vi "Required Buffer Size.vi"(8 "error in (no error)":errorcluster, 11 "Transfer Configuration in":refnum<class "Transfer Configuration.lvclass">) -> (0 "error out":errorcluster, 2 "required buffer size":u64 format="%d bytes", 3 "Transfer Configuration out":refnum<class "Transfer Configuration.lvclass">)   [LabVIEW 2017, in "DSF Core.lvlib" / "Transfer Configuration.lvclass"]
uses:
  Transfer Configuration.lvclass
  Transfer Configuration.lvclass/Transfer Configuration.ctl
  Shared/VIs/Sizeof.vi
  DSF Core.lvlib
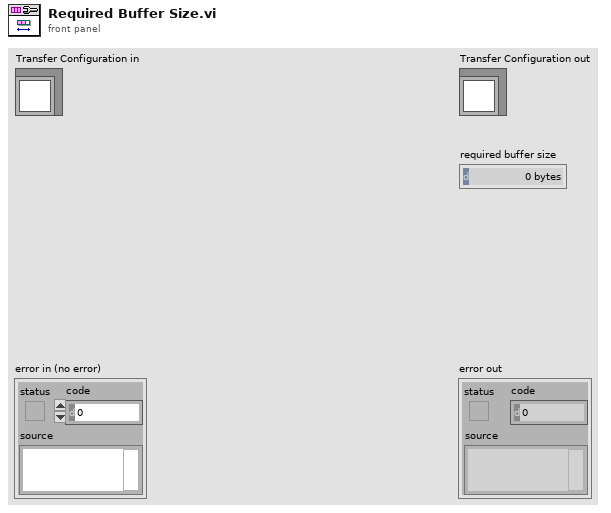
[diagram p1: front panel]
types:
  T1 = typedef "DSF Core.lvlib/DSF Engine Channel Configuration.ctl" = cluster{"engine offset":u64, "name":string, "data type":T2, "count":u64, "buffer offset":u64}
  T2 = typedef "DSF Core.lvlib/DSF Data Type.ctl" = enum8{"Bool", "SGL", "DBL", "I8", "I16", "I32", "I64", "U8", "U16", "U32", "U64"}
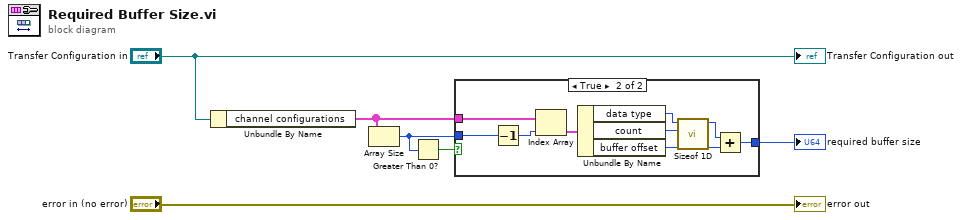
[diagram p0: block diagram]
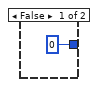
[diagram p2: hidden frame]
diagram:
  n1 = Unbundle By Name("Transfer Configuration in") -> ("channel configurations"=w4:T1[])
  n2 = Array Size(array=w4) -> (size(s)=w6:i32)
  n3 = Greater Than 0?(x=w6) -> (x > 0?=w5:bool)
  n4 = case shown="True" w5 {
    tunnel: w6 -> [_ w16]
    tunnel: w4 -> [_ w15]
    tunnel: [u64 0 w8] -> w2
    frame False {
    }
    frame True {
      n5 = Decrement(x=w16) -> (x-1=w14:i32)
      n6 = Index Array(array=w15, index=w14) -> (element=w13:T1)
      n7 = Unbundle By Name(w13) -> ("data type"=w12:T2, "count"=w11:u64, "buffer offset"=w10:u64)
      n8 = call "Sizeof 1D.vi"("count"=w11, "data type"=w12) -> ("size in bytes"=w9:u64)  [unwired: 9 in]
      n9 = Add(x=w9, y=w10) -> (x+y=w8:u64)
    }
  }
  "required buffer size" <- w2
  "error out" <- "error in (no error)"
  "Transfer Configuration out" <- "Transfer Configuration in"
